vi "H5Tenum_valueof (U16).vi"(6 "error in (no error)":errorcluster, 7 "Default Value":u16, 8 "String":string, 9 "HDF5 Type Ref":T1) -> (0 "error out":errorcluster, 1 "Member Value":u16, 3 "HDF5 Type Ref out":T1)   [LabVIEW 2017]
doc: "Returns the value corresponding to a specified member \n of an enumeration datatype."
uses:
  <vilib>/UPVI/lvhdf5/library.llb/HDF5 Ref.ctl
  <vilib>/UPVI/lvhdf5/hdf5.dll
panel:
  # "LVHDF5 Toolkit\nCopyright (c) 2005-2013 by Jason D. Sommerville\nCopyright (c) 2014 by UPVI, LLC.\n\nThis use and distribution of this file is governed by the terms found in \nLICENSE.txt distributed with this toolkit and installed at\n <user.lib>\\_lvhdf5\\LICENSE.txt"
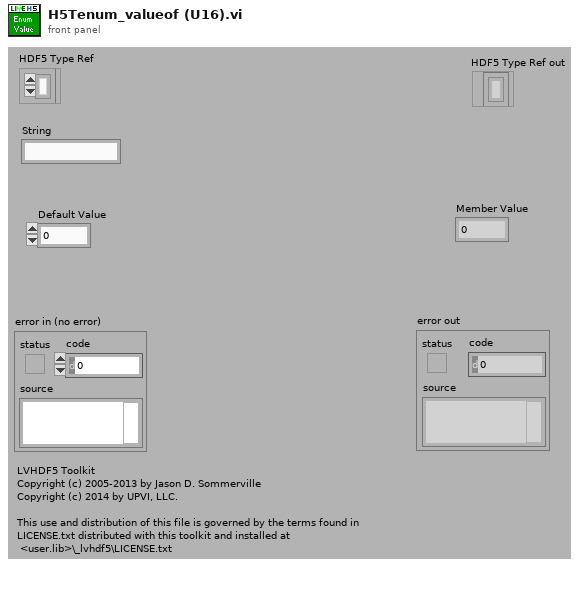
[diagram p1: front panel]
types:
  T1 = typedef "HDF5 Ref.ctl" = refnum<k1>
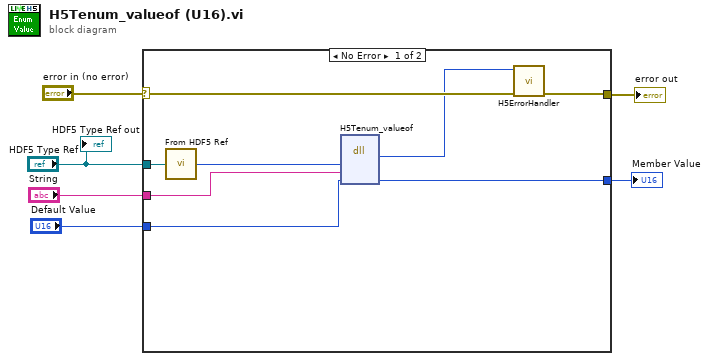
[diagram p0: block diagram]
diagram:
  n1 = case shown="No Error" "error in (no error)" {
    selector: "error in (no error)" -> [w14 w16]
    tunnel: [w13 w16] -> w5
    tunnel: "HDF5 Type Ref" -> [w11 _]
    tunnel: "String" -> [w8 _]
    tunnel: [w9 w15] -> w2
    tunnel: "Default Value" -> [w7 w15]
    frame No Error {
      n2 = call <vilib>:"From HDF5 Ref.vi"("HDF5 Ref"=w11) -> ("I32"=w10:i32)
      n3 = dll-call lib="C:/Program Files/National Instruments/LabVIEW 2017/vi.lib/UPVI/lvhdf5/hdf5.dll" fn="H5Tenum_valueof"("type_id"=w10, "name"=w8, "value"=w7) -> ("return type"=w12:i32, "value"=w9:u16)  [unwired: 5 in, 2 out]
      n4 = call <vilib>:"H5ErrorHandler.vi"("error in (no error)"=w14, "herr_t"=w12) -> ("error out"=w13:errorcluster)  [unwired: 3 in, 4 out]
    }
    frame Error {
    }
  }
  "error out" <- w5
  "Member Value" <- w2
  "HDF5 Type Ref out" <- "HDF5 Type Ref"
